vi "Test.vi"(8 "error in (no error)":errorcluster) -> (0 "error out":errorcluster)   [LabVIEW 2018]
panel:
  out "x+y":dbl
  in  "Numeric 2":dbl
  in  "Numeric":dbl
  # "Changes made for branch\nChanged in Branch"
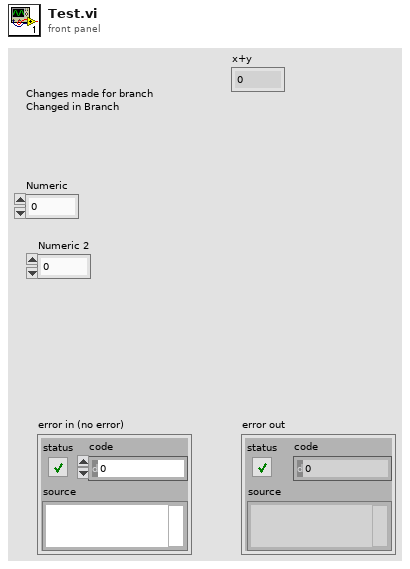
[diagram p1: front panel]
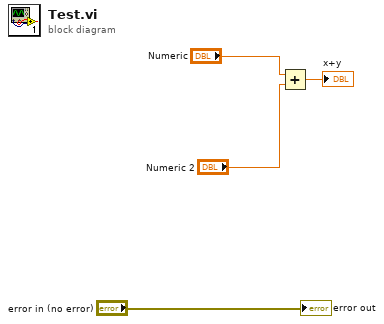
[diagram p0: block diagram]
diagram:
  n1 = Add(x="Numeric", y="Numeric 2") -> (x+y=→"x+y":dbl)
  "error out" <- "error in (no error)"
